vi "getStatusFlagsAllAxis.vi"(8 "error":errorcluster, 11 "connection ID":refnum<k5>) -> (0 "error out":errorcluster, 2 "Output parameters":T1, 3 "connection ID out":refnum<k5>)   [LabVIEW 2016, in "amc_api.lvlib"]
doc: "This function returns several status flags of all three axes"
uses:
  amc_api.lvlib
panel:
  out "jsonRespIn":string
  out "JSON-response":string="{\"jsonrpc\":\"2.0\",\"method\":\"\",\"params\":[5,1.245,true,\"name\"],\"id\":\"1\"}"
  out "JSON request":string
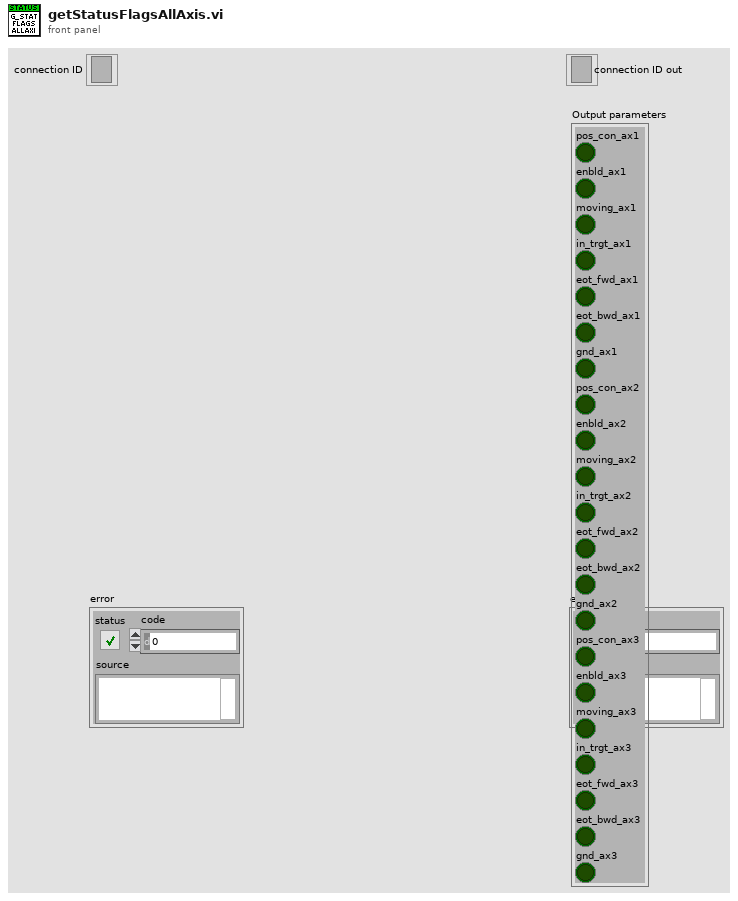
[diagram p1: front panel]
types:
  T1 = cluster{"pos_con_ax1":bool, "enbld_ax1":bool, "moving_ax1":bool, "in_trgt_ax1":bool, "eot_fwd_ax1":bool, "eot_bwd_ax1":bool, "gnd_ax1":bool, "pos_con_ax2":bool, "enbld_ax2":bool, "moving_ax2":bool, "in_trgt_ax2":bool, "eot_fwd_ax2":bool, "eot_bwd_ax2":bool, "gnd_ax2":bool, "pos_con_ax3":bool, "enbld_ax3":bool, "moving_ax3":bool, "in_trgt_ax3":bool, "eot_fwd_ax3":bool, "eot_bwd_ax3":bool, "gnd_ax3":bool}
  T2 = cluster{"jsonrpc":string, "method":string, "params":string[], "id":string, "api":i32, "pid":string}
  T3 = enum16{"Standard", "Buffered", "CRLF", "Immediate"}
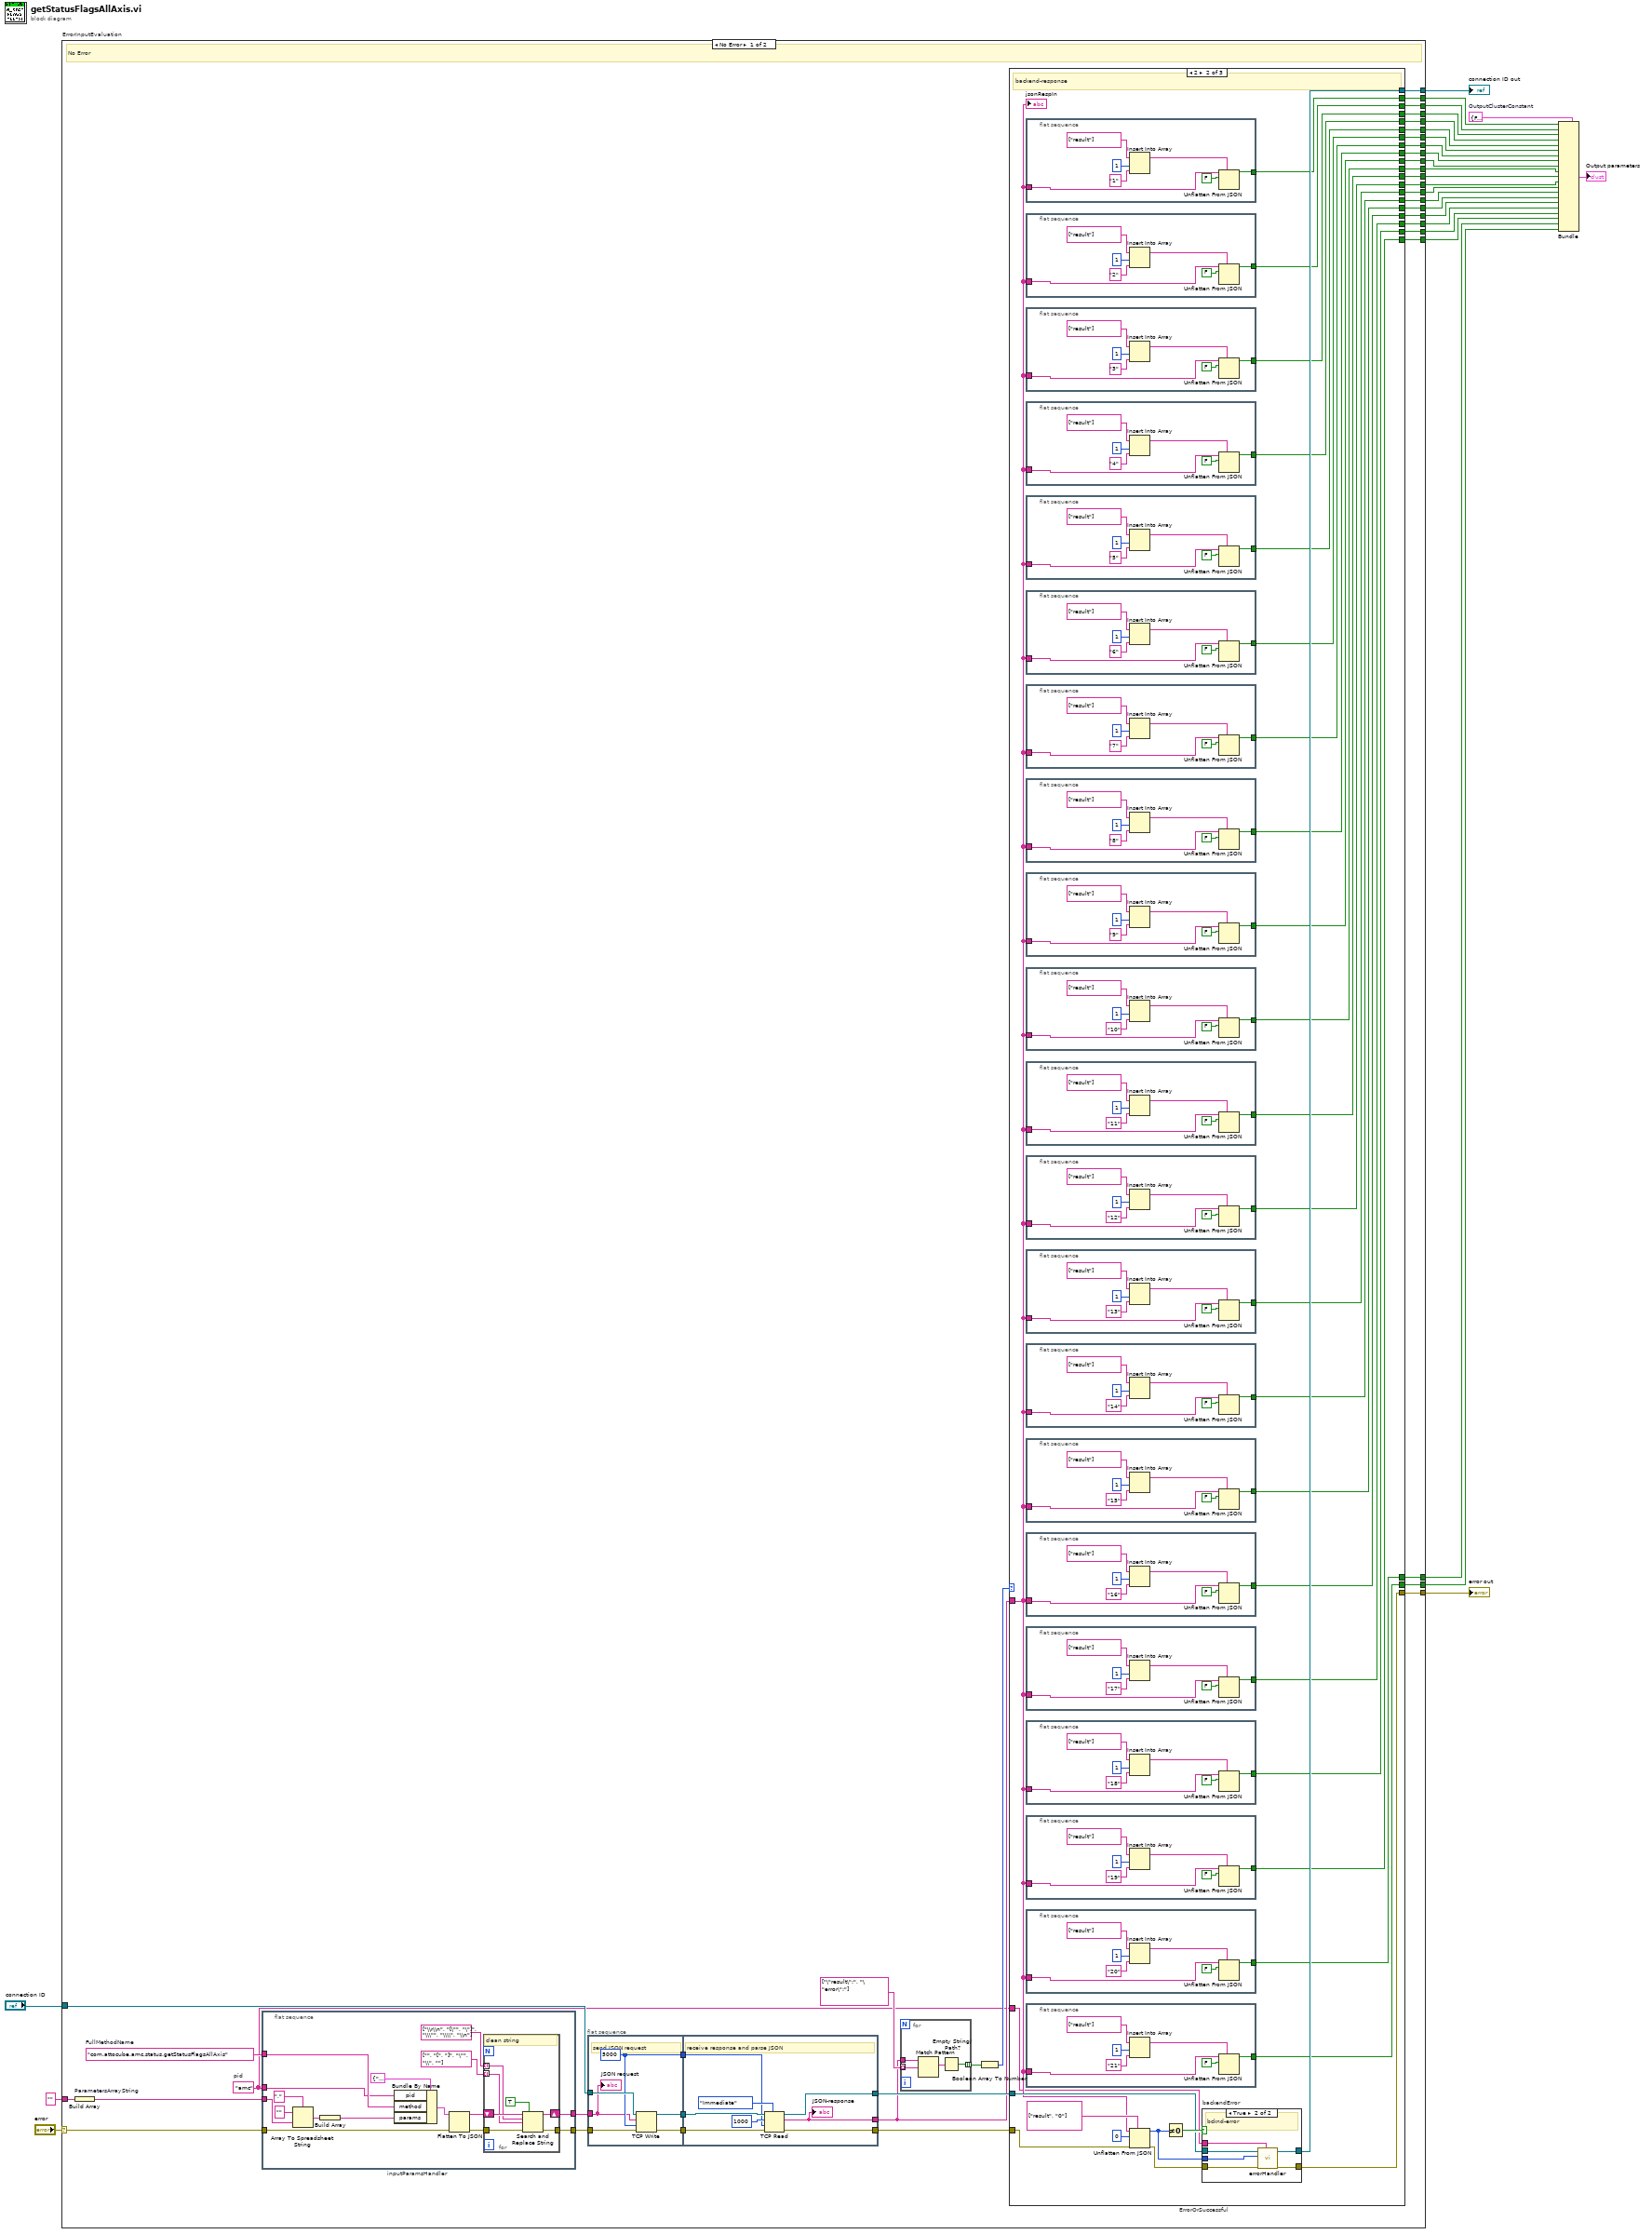
[diagram p0: block diagram]
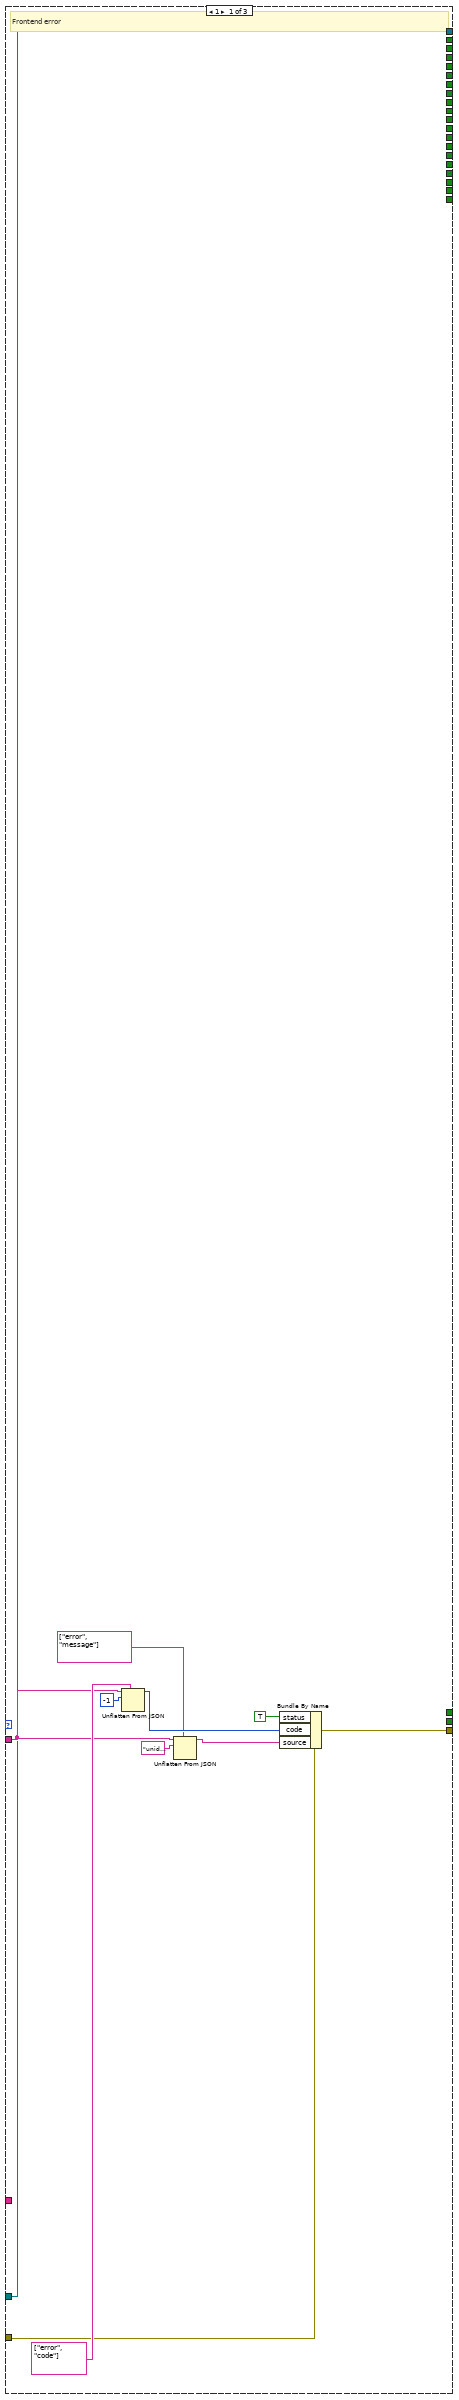
[diagram p2: hidden frame]
diagram:
  w27 = T1 {"pos_con_ax1"=FALSE, "enbld_ax1"=FALSE, "moving_ax1"=FALSE, "in_trgt_ax1"=FALSE, "eot_fwd_ax1"=FALSE, "eot_bwd_ax1"=FALSE, "gnd_ax1"=FALSE, "pos_con_ax2"=FALSE, "enbld_ax2"=FALSE, "moving_ax2"=FALSE, "in_trgt_ax2"=FALSE, "eot_fwd_ax2"=FALSE, "eot_bwd_ax2"=FALSE, "gnd_ax2"=FALSE, "pos_con_ax3"=FALSE, "enbld_ax3"=FALSE, "moving_ax3"=FALSE, "in_trgt_ax3"=FALSE, "eot_fwd_ax3"=FALSE, "eot_bwd_ax3"=FALSE, "gnd_ax3"=FALSE}  # OutputClusterConstant
  n1 = case "ErrorInputEvaluation" shown="No Error" "error" {
    selector: "error" -> [w55 w310]
    tunnel: "connection ID" -> [w65 w311]
    tunnel: [w57 w310] -> w26
    tunnel: [w58 w311] -> w25
    tunnel: "" -> [w50 _]
    tunnel: [w49 _] -> w22
    tunnel: [w48 _] -> w21
    tunnel: [w47 _] -> w20
    tunnel: [w46 _] -> w19
    tunnel: [w45 _] -> w18
    tunnel: [w44 _] -> w17
    tunnel: [w43 _] -> w16
    tunnel: [w42 _] -> w15
    tunnel: [w41 _] -> w14
    tunnel: [w40 _] -> w13
    tunnel: [w39 _] -> w12
    tunnel: [w38 _] -> w11
    tunnel: [w37 _] -> w10
    tunnel: [w36 _] -> w9
    tunnel: [w35 _] -> w8
    tunnel: [w34 _] -> w7
    tunnel: [w33 _] -> w6
    tunnel: [w32 _] -> w5
    tunnel: [w31 _] -> w4
    tunnel: [w30 _] -> w3
    tunnel: [w29 _] -> w2
    frame No Error {
      w51 = "amc"  # pid
      w56 = "com.attocube.amc.status.getStatusFlagsAllAxis"  # FullMethodName
      # "No Error"
      n2 = Build Array "ParametersArrayString"(w50) -> (w54:string[])
      n3 = flat-sequence "inputParamsHandler" {
        tunnel: [w74] -> w53
        tunnel: w54 -> [w80]
        tunnel: w55 -> [w79]
        tunnel: [w76] -> w52
        tunnel: w56 -> [w70]
        tunnel: w51 -> [w69]
        frame #0 {
          n4 = Array To Spreadsheet String(delimiter (Tab)=",", array=w80, 3:"" ("format string")) -> (spreadsheet string=w82:string)
          n5 = Build Array "Build Array"(w82) -> (w71:string[])
          n6 = Bundle By Name(cluster=T2 {"jsonrpc"="2.0", "method"="com.attocube.amc.res.setRESReadOutFreq", "params"=[], "id"="1", "api"=2, "pid"=""}, "pid"=w69, "method"=w70, "params"=w71) -> (w81:T2)
          n7 = Flatten To JSON(anything=w81, error in (no error)=w79) -> (JSON string=w75:string, 11:w77:errorcluster)  [unwired: 1 in]
          n8 = for {
            tunnel: string[] ["\\r\\n", "[\"", "\"]", "\\\"", "\\\\", "\\n"] ("search string") -> [w88] mode=indexing
            tunnel: string[] ["", "[", "]", "\"", "\\", ""] ("replace string (\"\")") -> [w87] mode=indexing
            shift-right: [w90] -> w74
            shift-left: w75 -> [w89]
            tunnel: w77 -> [w86]
            tunnel: [w85] -> w76
            # "clean string"
            n9 = Search and Replace String(replace all?=TRUE ("replace all? (F)"), input string=w89, search string=w88, replace string=w87, error in=w86) -> (result string=w90:string, error out=w85:errorcluster)  [unwired: 3 in, 2 out]
          }
        }
      }
      n10 = flat-sequence {
        tunnel: w65 -> [w301]
        tunnel: [w299] -> w68
        tunnel: [w300] -> w67
        tunnel: w52 -> [w296]
        tunnel: [w298] -> w66
        tunnel: w53 -> [w297]
        tunnel: [w305] -> w61
        tunnel: w68 -> [w307]
        tunnel: w67 -> [w306]
        tunnel: [w303] -> w60
        tunnel: w66 -> [w304]
        tunnel: [w302] -> w59
        frame #0 {
          w298 = 5000 ("timeout ms (25000)")
          # "send JSON request"
          n11 = TCP Write(connection ID=w301, data in=w297, error in (no error)=w296, 9:w298) -> (connection ID out=w299:refnum<k5>, error out=w300:errorcluster)  [unwired: 1 out]
          "JSON request" <- w297
        }
        frame #1 {
          # "receive response and parse JSON"
          n12 = TCP Read(connection ID=w307, bytes to read=1000, error in (no error)=w306, 7:T3."Immediate" ("mode (standard)"), 9:w304) -> (connection ID out=w305:refnum<k5>, data out=w302:string, error out=w303:errorcluster)
          "JSON-response" <- w302
        }
      }
      n13 = for {
        tunnel: string[] ["\"result\":", "\"error\":"] ("path") -> [w94] mode=indexing
        tunnel: [w92] -> w63 mode=indexing
        tunnel: w59 -> [w95]
        n14 = Match Pattern(string=w95, regular expression=w94) -> (match substring=w93:string)  [unwired: 1 in, 3 out]
        n15 = Empty String/Path?(string/path=w93) -> (empty?=w92:bool)
      }
      n16 = Boolean Array To Number(Boolean array=w63) -> (number=w62:u32)
      n17 = case "ErrorOrSuccessful" shown="2" w62 {
        tunnel: w59 -> [w98 w129 _]
        tunnel: w61 -> [w96 w132 w295]
        tunnel: [w96 w131 w295] -> w58
        tunnel: [w99 w130 w294] -> w57
        tunnel: w60 -> [w97 w133 w294]
        tunnel: w51 -> [_ w128 _]
        tunnel: [_ w127 _] -> w49
        tunnel: [_ w126 _] -> w48
        tunnel: [_ w125 _] -> w47
        tunnel: [_ w124 _] -> w46
        tunnel: [_ w123 _] -> w45
        tunnel: [_ w122 _] -> w44
        tunnel: [_ w121 _] -> w43
        tunnel: [_ w120 _] -> w42
        tunnel: [_ w119 _] -> w41
        tunnel: [_ w118 _] -> w40
        tunnel: [_ w117 _] -> w39
        tunnel: [_ w116 _] -> w38
        tunnel: [_ w115 _] -> w37
        tunnel: [_ w114 _] -> w36
        tunnel: [_ w113 _] -> w35
        tunnel: [_ w112 _] -> w34
        tunnel: [_ w111 _] -> w33
        tunnel: [_ w110 _] -> w32
        tunnel: [_ w109 _] -> w31
        tunnel: [_ w108 _] -> w30
        tunnel: [_ w107 _] -> w29
        frame 1 {
          # "Frontend error"
          n18 = Unflatten From JSON(path=string[] ["error", "code"], JSON string=w98, type and defaults=-1) -> (value=w105:i32)  [unwired: 4 in, 1 out]
          n19 = Unflatten From JSON(path=string[] ["error", "message"], JSON string=w98, type and defaults="unidentified error") -> (value=w106:string)  [unwired: 4 in, 1 out]
          n20 = Bundle By Name(cluster=w97, "status"=TRUE, "code"=w105, "source"=w106) -> (w99:errorcluster)
        }
        frame 2 {
          # "backend-response"
          n21 = flat-sequence "out_bool" {
            tunnel: w129 -> [w284]
            tunnel: [w279] -> w127
            frame #0 {
              n22 = Insert Into Array "Insert Into Array"(array=string[] ["result"] ("path"), index=1, new element="1" ("idx")) -> (w281:string[])
              n23 = Unflatten From JSON(path=w281, JSON string=w284, type and defaults=FALSE) -> (value=w279:bool)  [unwired: 4 in, 1 out]
            }
          }
          n24 = flat-sequence "out_bool" {
            tunnel: w129 -> [w277]
            tunnel: [w272] -> w126
            frame #0 {
              n25 = Insert Into Array "Insert Into Array"(array=string[] ["result"] ("path"), index=1, new element="2" ("idx")) -> (w274:string[])
              n26 = Unflatten From JSON(path=w274, JSON string=w277, type and defaults=FALSE) -> (value=w272:bool)  [unwired: 4 in, 1 out]
            }
          }
          n27 = flat-sequence "out_bool" {
            tunnel: w129 -> [w270]
            tunnel: [w265] -> w125
            frame #0 {
              n28 = Insert Into Array "Insert Into Array"(array=string[] ["result"] ("path"), index=1, new element="3" ("idx")) -> (w267:string[])
              n29 = Unflatten From JSON(path=w267, JSON string=w270, type and defaults=FALSE) -> (value=w265:bool)  [unwired: 4 in, 1 out]
            }
          }
          n30 = flat-sequence "out_bool" {
            tunnel: w129 -> [w263]
            tunnel: [w258] -> w124
            frame #0 {
              n31 = Insert Into Array "Insert Into Array"(array=string[] ["result"] ("path"), index=1, new element="4" ("idx")) -> (w260:string[])
              n32 = Unflatten From JSON(path=w260, JSON string=w263, type and defaults=FALSE) -> (value=w258:bool)  [unwired: 4 in, 1 out]
            }
          }
          n33 = flat-sequence "out_bool" {
            tunnel: w129 -> [w256]
            tunnel: [w251] -> w123
            frame #0 {
              n34 = Insert Into Array "Insert Into Array"(array=string[] ["result"] ("path"), index=1, new element="5" ("idx")) -> (w253:string[])
              n35 = Unflatten From JSON(path=w253, JSON string=w256, type and defaults=FALSE) -> (value=w251:bool)  [unwired: 4 in, 1 out]
            }
          }
          n36 = flat-sequence "out_bool" {
            tunnel: w129 -> [w249]
            tunnel: [w244] -> w122
            frame #0 {
              n37 = Insert Into Array "Insert Into Array"(array=string[] ["result"] ("path"), index=1, new element="6" ("idx")) -> (w246:string[])
              n38 = Unflatten From JSON(path=w246, JSON string=w249, type and defaults=FALSE) -> (value=w244:bool)  [unwired: 4 in, 1 out]
            }
          }
          n39 = flat-sequence "out_bool" {
            tunnel: w129 -> [w242]
            tunnel: [w237] -> w121
            frame #0 {
              n40 = Insert Into Array "Insert Into Array"(array=string[] ["result"] ("path"), index=1, new element="7" ("idx")) -> (w239:string[])
              n41 = Unflatten From JSON(path=w239, JSON string=w242, type and defaults=FALSE) -> (value=w237:bool)  [unwired: 4 in, 1 out]
            }
          }
          n42 = flat-sequence "out_bool" {
            tunnel: w129 -> [w235]
            tunnel: [w230] -> w120
            frame #0 {
              n43 = Insert Into Array "Insert Into Array"(array=string[] ["result"] ("path"), index=1, new element="8" ("idx")) -> (w232:string[])
              n44 = Unflatten From JSON(path=w232, JSON string=w235, type and defaults=FALSE) -> (value=w230:bool)  [unwired: 4 in, 1 out]
            }
          }
          n45 = flat-sequence "out_bool" {
            tunnel: w129 -> [w228]
            tunnel: [w223] -> w119
            frame #0 {
              n46 = Insert Into Array "Insert Into Array"(array=string[] ["result"] ("path"), index=1, new element="9" ("idx")) -> (w225:string[])
              n47 = Unflatten From JSON(path=w225, JSON string=w228, type and defaults=FALSE) -> (value=w223:bool)  [unwired: 4 in, 1 out]
            }
          }
          n48 = flat-sequence "out_bool" {
            tunnel: w129 -> [w221]
            tunnel: [w216] -> w118
            frame #0 {
              n49 = Insert Into Array "Insert Into Array"(array=string[] ["result"] ("path"), index=1, new element="10" ("idx")) -> (w218:string[])
              n50 = Unflatten From JSON(path=w218, JSON string=w221, type and defaults=FALSE) -> (value=w216:bool)  [unwired: 4 in, 1 out]
            }
          }
          n51 = flat-sequence "out_bool" {
            tunnel: w129 -> [w214]
            tunnel: [w209] -> w117
            frame #0 {
              n52 = Insert Into Array "Insert Into Array"(array=string[] ["result"] ("path"), index=1, new element="11" ("idx")) -> (w211:string[])
              n53 = Unflatten From JSON(path=w211, JSON string=w214, type and defaults=FALSE) -> (value=w209:bool)  [unwired: 4 in, 1 out]
            }
          }
          n54 = flat-sequence "out_bool" {
            tunnel: w129 -> [w207]
            tunnel: [w202] -> w116
            frame #0 {
              n55 = Insert Into Array "Insert Into Array"(array=string[] ["result"] ("path"), index=1, new element="12" ("idx")) -> (w204:string[])
              n56 = Unflatten From JSON(path=w204, JSON string=w207, type and defaults=FALSE) -> (value=w202:bool)  [unwired: 4 in, 1 out]
            }
          }
          n57 = flat-sequence "out_bool" {
            tunnel: w129 -> [w200]
            tunnel: [w195] -> w115
            frame #0 {
              n58 = Insert Into Array "Insert Into Array"(array=string[] ["result"] ("path"), index=1, new element="13" ("idx")) -> (w197:string[])
              n59 = Unflatten From JSON(path=w197, JSON string=w200, type and defaults=FALSE) -> (value=w195:bool)  [unwired: 4 in, 1 out]
            }
          }
          n60 = flat-sequence "out_bool" {
            tunnel: w129 -> [w193]
            tunnel: [w188] -> w114
            frame #0 {
              n61 = Insert Into Array "Insert Into Array"(array=string[] ["result"] ("path"), index=1, new element="14" ("idx")) -> (w190:string[])
              n62 = Unflatten From JSON(path=w190, JSON string=w193, type and defaults=FALSE) -> (value=w188:bool)  [unwired: 4 in, 1 out]
            }
          }
          n63 = flat-sequence "out_bool" {
            tunnel: w129 -> [w186]
            tunnel: [w181] -> w113
            frame #0 {
              n64 = Insert Into Array "Insert Into Array"(array=string[] ["result"] ("path"), index=1, new element="15" ("idx")) -> (w183:string[])
              n65 = Unflatten From JSON(path=w183, JSON string=w186, type and defaults=FALSE) -> (value=w181:bool)  [unwired: 4 in, 1 out]
            }
          }
          n66 = flat-sequence "out_bool" {
            tunnel: w129 -> [w179]
            tunnel: [w174] -> w112
            frame #0 {
              n67 = Insert Into Array "Insert Into Array"(array=string[] ["result"] ("path"), index=1, new element="16" ("idx")) -> (w176:string[])
              n68 = Unflatten From JSON(path=w176, JSON string=w179, type and defaults=FALSE) -> (value=w174:bool)  [unwired: 4 in, 1 out]
            }
          }
          n69 = flat-sequence "out_bool" {
            tunnel: w129 -> [w172]
            tunnel: [w167] -> w111
            frame #0 {
              n70 = Insert Into Array "Insert Into Array"(array=string[] ["result"] ("path"), index=1, new element="17" ("idx")) -> (w169:string[])
              n71 = Unflatten From JSON(path=w169, JSON string=w172, type and defaults=FALSE) -> (value=w167:bool)  [unwired: 4 in, 1 out]
            }
          }
          n72 = flat-sequence "out_bool" {
            tunnel: w129 -> [w165]
            tunnel: [w160] -> w110
            frame #0 {
              n73 = Insert Into Array "Insert Into Array"(array=string[] ["result"] ("path"), index=1, new element="18" ("idx")) -> (w162:string[])
              n74 = Unflatten From JSON(path=w162, JSON string=w165, type and defaults=FALSE) -> (value=w160:bool)  [unwired: 4 in, 1 out]
            }
          }
          n75 = flat-sequence "out_bool" {
            tunnel: w129 -> [w158]
            tunnel: [w153] -> w109
            frame #0 {
              n76 = Insert Into Array "Insert Into Array"(array=string[] ["result"] ("path"), index=1, new element="19" ("idx")) -> (w155:string[])
              n77 = Unflatten From JSON(path=w155, JSON string=w158, type and defaults=FALSE) -> (value=w153:bool)  [unwired: 4 in, 1 out]
            }
          }
          n78 = flat-sequence "out_bool" {
            tunnel: w129 -> [w151]
            tunnel: [w146] -> w108
            frame #0 {
              n79 = Insert Into Array "Insert Into Array"(array=string[] ["result"] ("path"), index=1, new element="20" ("idx")) -> (w148:string[])
              n80 = Unflatten From JSON(path=w148, JSON string=w151, type and defaults=FALSE) -> (value=w146:bool)  [unwired: 4 in, 1 out]
            }
          }
          n81 = flat-sequence "out_bool" {
            tunnel: w129 -> [w144]
            tunnel: [w139] -> w107
            frame #0 {
              n82 = Insert Into Array "Insert Into Array"(array=string[] ["result"] ("path"), index=1, new element="21" ("idx")) -> (w141:string[])
              n83 = Unflatten From JSON(path=w141, JSON string=w144, type and defaults=FALSE) -> (value=w139:bool)  [unwired: 4 in, 1 out]
            }
          }
          n84 = Unflatten From JSON(path=string[] ["result", "0"], JSON string=w129, type and defaults=0, error in (no error)=w133) -> (value=w138:i32, error out=w136:errorcluster)  [unwired: 3 in]
          n85 = Not Equal To 0?(x=w138) -> (x != 0?=w137:bool)
          n86 = case "backendError" shown="True" w137 {
            tunnel: w138 -> [_ w293]
            tunnel: w136 -> [w287 w292]
            tunnel: [w286 w291] -> w131
            tunnel: [w287 w290] -> w130
            tunnel: w132 -> [w286 w289]
            tunnel: w128 -> [_ w288]
            frame False {
              # "successful"
            }
            frame True {
              # "bcknd-error"
              n87 = call "errorHandler.vi"("pid"=w288, "error in"=w292, "errNbr"=w293, "connection ID"=w289) -> ("error out 2"=w290:errorcluster, "connection ID out"=w291:refnum<k5>)  [unwired: 6 in]
            }
          }
          "jsonRespIn" <- w129
        }
        frame Default {
          # "NoResponse"
        }
      }
    }
    frame Error {
      # "Error"
    }
  }
  "error out" <- w26
  "connection ID out" <- w25
  n88 = Bundle ("BundleOutputs")(cluster=w27, "pos_con_ax1"=w22, "enbld_ax1"=w21, "moving_ax1"=w20, "in_trgt_ax1"=w19, "eot_fwd_ax1"=w18, "eot_bwd_ax1"=w17, "gnd_ax1"=w16, "pos_con_ax2"=w15, "enbld_ax2"=w14, "moving_ax2"=w13, "in_trgt_ax2"=w12, "eot_fwd_ax2"=w11, "eot_bwd_ax2"=w10, "gnd_ax2"=w9, "pos_con_ax3"=w8, "enbld_ax3"=w7, "moving_ax3"=w6, "in_trgt_ax3"=w5, "eot_fwd_ax3"=w4, "eot_bwd_ax3"=w3, "gnd_ax3"=w2) -> (→"Output parameters":T1)
